vi "auth.vi"(8 "signature":string="signature", 11 "access_key":string) -> (3 "auth":string)   [LabVIEW 2019]
panel:
  out "concatenated string":string
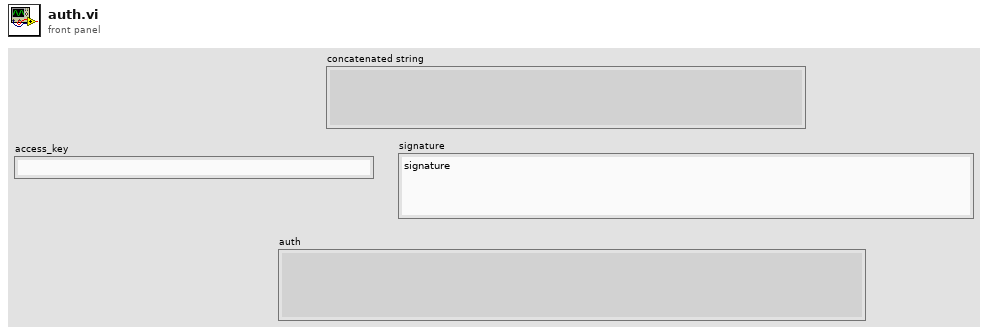
[diagram p1: front panel]
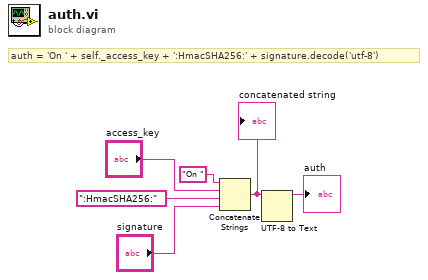
[diagram p0: block diagram]
diagram:
  # "auth = 'On ' + self._access_key + ':HmacSHA256:' + signature.decode('utf-8')"
  n1 = Concatenate Strings("On ", "access_key", ":HmacSHA256:" ("string"), "signature") -> (w2:string)
  "concatenated string" <- w2
  n2 = UTF-8 to Text(11:w2) -> (3:→"auth":string)  [unwired: 2 in, 1 out]
